vi "Set Target Attacker.vi"(7 "GOAL":dbl[](array[numeric]), 9 "Position":dbl[](array[numeric]), 11 "Target":dbl[](array[numeric])) -> (1 "output":dbl[](array[numeric]))   [LabVIEW 2016]
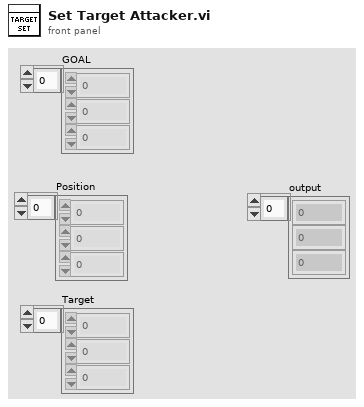
[diagram p1: front panel]
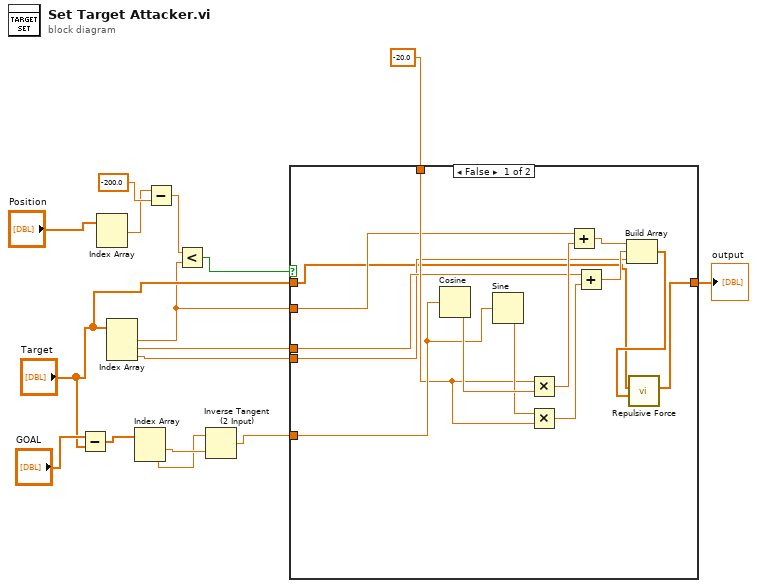
[diagram p0: block diagram]
diagram:
  n1 = Subtract(x="GOAL", y="Target") -> (x-y=w13:dbl[])
  n2 = Index Array(array="Position") -> (element #1=w2:dbl)  [unwired: 2 in, 1 out]
  n3 = Index Array(array="Target") -> (element #1=w7:dbl, element #2=w6:dbl, element #3=w5:dbl)  [unwired: 3 in]
  n4 = Index Array(array=w13) -> (element #1=w12:dbl, element #2=w11:dbl)  [unwired: 2 in]
  n5 = Subtract(x=w2, y=-200.0) -> (x-y=w1:dbl)
  n6 = Less?(x=w1, y=w7) -> (x < y?=w16:bool)
  n7 = Inverse Tangent (2 Input)(1:w12, 2:w11) -> (0:w8:dbl)
  n8 = case shown="False" w16 {
    tunnel: [w17 w31] -> w15
    tunnel: "Target" -> [w18 w31]
    tunnel: w8 -> [w28 _]
    tunnel: -20.0 -> [w27 _]
    tunnel: w7 -> [w26 _]
    tunnel: w6 -> [w24 _]
    tunnel: w5 -> [w20 _]
    frame False {
      n9 = Cosine(x=w28) -> (cos(x)=w30:dbl)
      n10 = Sine(x=w28) -> (sin(x)=w29:dbl)
      n11 = Multiply(x=w27, y=w30) -> (x*y=w25:dbl)
      n12 = Multiply(x=w29, y=w27) -> (x*y=w23:dbl)
      n13 = Add(x=w26, y=w25) -> (x+y=w22:dbl)
      n14 = Add(x=w24, y=w23) -> (x+y=w21:dbl)
      n15 = Build Array(w22, w21, w20) -> (w19:dbl[])
      n16 = call "Repulsive Force.vi"("Target"=w19, "Robot Position"=w18) -> ("out"=w17:dbl[])  [unwired: 9 in]
    }
    frame True {
    }
  }
  "output" <- w15
